vi "Name FIFOs Top.vi"(8 "error in (no error)":errorcluster, 9 "Current Bus Number":i32, 10 "Device Channels":i32[](array[numeric]), 11 "Curent Bus Path":path) -> (0 "error out":errorcluster)   [LabVIEW 2014, in "SPI Engine Scripting.lvlib"]
uses:
  SPI Engine Scripting.lvlib
  State Machine/Controls/Values for Naming.ctl
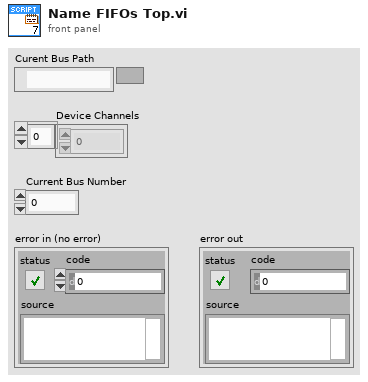
[diagram p1: front panel]
types:
  T1 = typedef "SPI Engine Scripting.lvlib/Values for Naming.ctl" = cluster{"Bus Number":i32, "Device Number":i32, "Channel Number":i32}
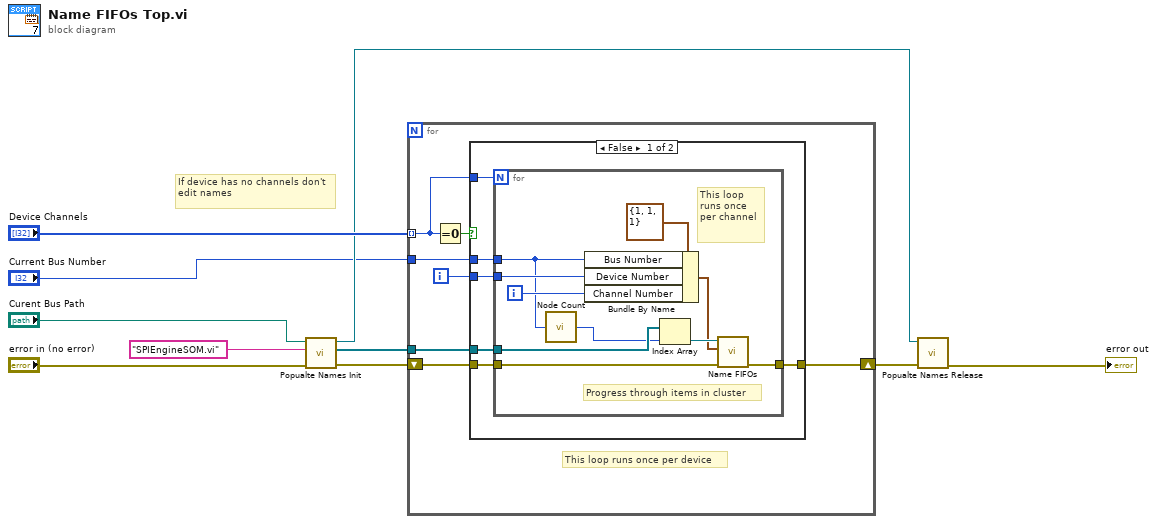
[diagram p0: block diagram]
diagram:
  # "If device has no channels don't edit names"
  n1 = call "Popualte Names Init.vi"("error in (no error)"="error in (no error)", "Engine Name"="SPIEngineSOM.vi" ("name or relative path"), "Destination Path"="Curent Bus Path") -> ("error out"=w4:errorcluster, "Communication FIFOs Elements"=w8:refnum<vi>[], "Communication FIFOs Refnum"=w6:refnum<vi>)  [unwired: 6 in]
  n2 = for {
    tunnel: w8 -> [w15]
    shift-right: [w16] -> w5
    shift-left: w4 -> [w17]
    tunnel: "Device Channels" -> [w11] mode=indexing
    tunnel: "Current Bus Number" -> [w12]
    i -> [w14]
    # "This loop runs once per device"
    n3 = Equal To 0?(x=w11) -> (x = 0?=w13:bool)
    n4 = case shown="False" w13 {
      tunnel: w17 -> [w23 w34]
      tunnel: [w22 w34] -> w16
      tunnel: w15 -> [w21 _]
      tunnel: w14 -> [w20 _]
      tunnel: w11 -> [w19 _]
      tunnel: w12 -> [w18 _]
      frame False {
        n5 = for {
          N: w19 -> [_]
          tunnel: [w33] -> w22
          tunnel: w23 -> [w32]
          tunnel: w21 -> [w31]
          tunnel: w20 -> [w27]
          tunnel: w18 -> [w25]
          i -> [w26]
          # "This loop runs once per channel"
          # "Progress through items in cluster"
          n6 = call "Node Count.vi"("Bus Number in"=w25) -> ("Node Number"=w24:i32)
          n7 = Bundle By Name(cluster=T1 {"Bus Number"=1, "Device Number"=1, "Channel Number"=1} ("Values for Naming"), "Bus Number"=w25, "Device Number"=w27, "Channel Number"=w26) -> (w29:T1)
          n8 = Index Array(array=w31, index=w24) -> (element=w30:refnum<vi>)
          n9 = call "Name FIFOs.vi"("error in (no error)"=w32, "Values for Naming"=w29, "Communications FIFOs Element"=w30) -> ("error out"=w33:errorcluster)  [unwired: 8 in]
        }
      }
      frame True {
      }
    }
  }
  n10 = call "Popualte Names Release.vi"("error in (no error)"=w5, "ClusterConstant in"=w6) -> ("error out"=→"error out":errorcluster)  [unwired: 9 in]
